vi "test Set Topology Updates Possible Connections.vi"(8 "error in (no error)":errorcluster, 11 "TestCase in":refnum<class "SLSC Switch Scripting Unit Tests.lvclass">) -> (0 "error out":errorcluster, 3 "TestCase out":refnum<class "SLSC Switch Scripting Unit Tests.lvclass">)   [LabVIEW 2017, in "SLSC Switch Scripting Unit Tests.lvclass"]
uses:
  SLSC Switch Scripting Unit Tests.lvclass
  <vilib>/addons/_JKI Toolkits/VI Tester/TestCase.llb/TestCase.lvclass
  NI-SWITCH Scripting.lvlib
  Properties/SLSC Switch All Properties.ctl
  Shared/Routing and Faulting Hardware API/Routing and Faulting Hardware API.lvlib
  Shared/Routing and Faulting Hardware API/Types/Possible Connections for Endpoint.ctl
  Custom Device/Find All SLSC Switch Custom Devices.vi
  C:/Program Files (x86)/National Instruments/LabVIEW 2017/vi.lib/addons/_JKI Toolkits/VI Tester/TestCase.llb/TestCase.lvclass
panel:
  in  "Save?":bool
  out "Output Filename":string
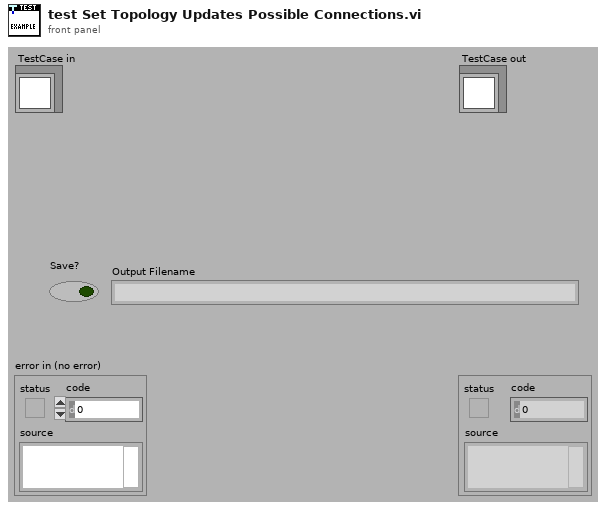
[diagram p1: front panel]
types:
  T1 = typedef "Routing and Faulting Hardware API.lvlib/Possible Connections for Endpoint.ctl" = cluster{"Source":string, "Destinations":string[]}
  T2 = typedef "NI-SWITCH Scripting.lvlib/SLSC Switch All Properties.ctl" = cluster{"Product Name":string, "Topology":string, "Switches JSON":string, "Description":string, "Reservation Group":string}
  T3 = typedef "Custom Device API.lvlib/Custom Device Item Ref.ctl" = u64
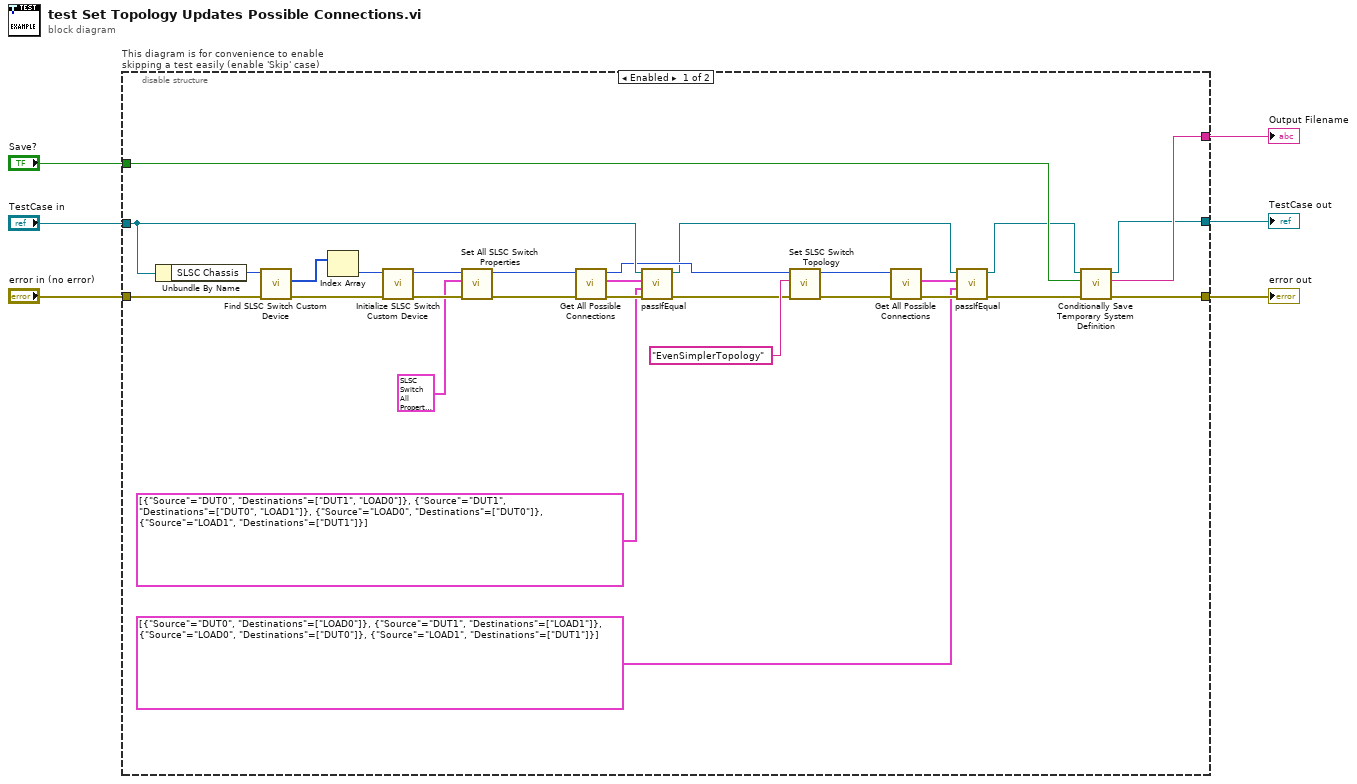
[diagram p0: block diagram]
diagram:
  n1 = disable-structure "This diagram is for convenience to enable skipping a test easily (enable 'Skip' case)" shown="Enabled" {
    disable-tunnel: "TestCase in" -> [w19 w39]
    disable-tunnel: [w33 w37] -> w3
    disable-tunnel: [w34 w38] -> w5
    disable-tunnel: "error in (no error)" -> [w27 w36]
    disable-tunnel: [w35 _] -> w2
    disable-tunnel: "Save?" -> [w32 _]
    frame Enabled {
      n2 = Unbundle By Name(w19) -> ("SLSC Chassis"=w28:u64)
      n3 = call-poly "Find SLSC Switch Custom Device.vi"("error in"=w27, "slsc chassis in"=w28) -> ("error out"=w30:errorcluster, "slsc switch custom devices"=w31:T3[])  [unwired: 7 in, 1 out]
      n4 = Index Array(array=w31) -> (element=w29:T3)  [unwired: 1 in]
      n5 = call "Initialize SLSC Switch Custom Device.vi"("error in"=w30, "slsc switch custom device in"=w29) -> ("error out"=w25:errorcluster, "slsc switch custom device out"=w26:T3)  [unwired: 7 in, 1 out]
      n6 = call "Set All SLSC Switch Properties.vi"("error in"=w25, "properties"=T2 {"Product Name"="Fake Device", "Topology"="SimpleTopology", "Switches JSON"="{\n   \"switchesSpecVersion\": 1,\n   \"relays\": [\n      {\n         \"name\": \"DUT0_LOAD0\",\n         \"actions\": [\n            {\n               \"type\": \"property\",\n               \"resource\": \"Foo\",\n               \"value\": \"Vendor.DUT0_LOAD0\"\n            },\n            {\n               \"type\": \"command\",\n               \"resource\": \"Foo\",\n               \"value\": \"Vendor.Update\"\n            }\n         ]\n      },\n      {\n         \"name\": \"DUT1_LOAD1\",\n         \"actions\": [\n            {\n               \"type\": \"property\",\n               \"resource\": \"Foo\",\n               \"value\": \"Vendor.DUT1_LOAD1\"\n            },\n            {\n               \"type\": \"command\",\n               \"resource\": \"Foo\",\n               \"value\": \"Vendor.Update\"\n            }\n         ]\n      },\n      {\n         \"name\": \"DUT0_DUT1\",\n         \"actions\": [\n            {\n               \"type\": \"property\",\n               \"resource\": \"Foo\",\n               \"value\": \"Vendor.DUT0_DUT1\"\n            },\n            {\n               \"type\": \"command\",\n               \"resource\": \"Foo\",\n               \"value\": \"Vendor.Update\"\n            }\n         ]\n      }\n   ],\n   \"topologies\": [\n      {\n         \"name\": \"SimpleTopology\",\n         \"initialState\": {\n            \"open\": [\n               \"DUT0_LOAD0\",\n               \"DUT1_LOAD1\",\n               \"DUT0_DUT1\"\n            ],\n            \"close\": []\n         },\n         \"channelList\": {\n            \"names\": [\n               \"DUT0\",\n               \"DUT1\",\n               \"LOAD0\",\n               \"LOAD1\"\n            ]\n         },\n         \"connectionList\": [\n            {\n               \"src\": \"DUT0\",\n               \"dest\": \"LOAD0\",\n               \"relays\": [\n                  \"DUT0_LOAD0\"\n               ]\n            },\n            {\n               \"src\": \"DUT1\",\n               \"dest\": \"LOAD1\",\n               \"relays\": [\n                  \"DUT1_LOAD1\"\n               ]\n            },\n            {\n               \"src\": \"DUT0\",\n               \"dest\": \"DUT1\",\n               \"relays\": [\n                  \"DUT0_DUT1\"\n               ]\n            }\n         ]\n      },\n      {\n         \"name\": \"EvenSimplerTopology\",\n         \"initialState\": {\n            \"open\": [\n               \"DUT0_LOAD0\",\n               \"DUT1_LOAD1\"\n            ],\n            \"close\": []\n         },\n         \"channelList\": {\n            \"names\": [\n               \"DUT0\",\n               \"DUT1\",\n               \"LOAD0\",\n               \"LOAD1\"\n            ]\n         },\n         \"connectionList\": [\n            {\n               \"src\": \"DUT0\",\n               \"dest\": \"LOAD0\",\n               \"relays\": [\n                  \"DUT0_LOAD0\"\n               ]\n            },\n            {\n               \"src\": \"DUT1\",\n               \"dest\": \"LOAD1\",\n               \"relays\": [\n                  \"DUT1_LOAD1\"\n               ]\n            }\n         ]\n      }\n   ],\n   \"multiStateRelays\": []\n}", "Description"="", "Reservation Group"=""} ("SLSC Switch All Properties"), "slsc switch custom device in"=w26) -> ("error out"=w22:errorcluster, "slsc switch custom device out"=w21:T3)  [unwired: 7 in]
      n7 = call "Get All Possible Connections.vi"("error in (no error)"=w22, "Hardware Ref in"=w21) -> ("error out"=w20:errorcluster, "Possible Connections"=w15:T1[], "Hardware Ref out"=w17:T3)  [unwired: 6 in, 1 out]
      n8 = call-dynamic "passIfEqual.vi"("error in (no error)"=w20, "y"=T1[] [{"Source"="DUT0", "Destinations"=["DUT1", "LOAD0"]}, {"Source"="DUT1", "Destinations"=["DUT0", "LOAD1"]}, {"Source"="LOAD0", "Destinations"=["DUT0"]}, {"Source"="LOAD1", "Destinations"=["DUT1"]}] ("Possible Connections"), "x"=w15, "TestCase in"=w19) -> ("error out"=w18:errorcluster, "TestCase out"=w10:refnum<class "SLSC Switch Scripting Unit Tests.lvclass">)  [unwired: 6 in]
      n9 = call "Set SLSC Switch Topology.vi"("error in"=w18, "topology"="EvenSimplerTopology" ("Topology"), "slsc switch custom device in"=w17) -> ("error out"=w12:errorcluster, "slsc switch custom device out"=w11:T3)  [unwired: 7 in]
      n10 = call "Get All Possible Connections.vi"("error in (no error)"=w12, "Hardware Ref in"=w11) -> ("error out"=w14:errorcluster, "Possible Connections"=w13:T1[])  [unwired: 6 in, 2 out]
      n11 = call-dynamic "passIfEqual.vi"("error in (no error)"=w14, "y"=T1[] [{"Source"="DUT0", "Destinations"=["LOAD0"]}, {"Source"="DUT1", "Destinations"=["LOAD1"]}, {"Source"="LOAD0", "Destinations"=["DUT0"]}, {"Source"="LOAD1", "Destinations"=["DUT1"]}] ("Possible Connections"), "x"=w13, "TestCase in"=w10) -> ("error out"=w8:errorcluster, "TestCase out"=w9:refnum<class "SLSC Switch Scripting Unit Tests.lvclass">)  [unwired: 6 in]
      n12 = call "Conditionally Save Temporary System Definition.vi"("error in (no error)"=w8, "Save?"=w32, "Test Case"=w9) -> ("error out"=w34:errorcluster, "filename"=w35:string, "Test Case"=w33:refnum<class "SLSC Switch Scripting Unit Tests.lvclass">)  [unwired: 6 in]
    }
    frame Disabled {
      # "skip test result while test is under development"
      n13 = call <vilib>:"skip.vi"("error in (no error)"=w36, "TestCase in"=w39) -> ("error out"=w38:errorcluster, "TestCase out"=w37:refnum<class "SLSC Switch Scripting Unit Tests.lvclass">)  [unwired: 8 in]
    }
  }
  "error out" <- w5
  "TestCase out" <- w3
  "Output Filename" <- w2
